vi "Get SMO RC Type.vi"(8 "error in (no error)":errorcluster, 11 "Inst.MagnetoInstrument in":refnum<class "Inst.Magneto.lvclass">) -> (0 "error out":errorcluster, 2 "Configuration.SMO.RC Type":T1=enum."STM", 3 "Inst.MagnetoInstrument out":refnum<class "Inst.Magneto.lvclass">)   [LabVIEW 2019, in "Inst.Magneto.lvclass"]
uses:
  Inst.Magneto.lvclass
  <userlib>/Levylab/Instrument Framework/SMOs/RemoteControl/Typedefs/RC Com Type--enum.ctl
  <userlib>/Levylab/Instrument Framework/Instrument Types/VSource/Instrument.VSource.lvclass
  <userlib>/Levylab/Instrument Framework/SMOs/RemoteControl/RemoteControl.lvclass
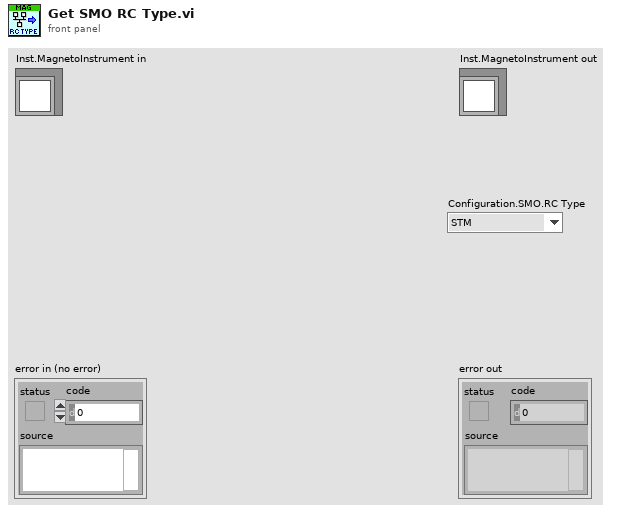
[diagram p1: front panel]
types:
  T1 = typedef "RemoteControl.lvclass/RC Com Type--enum.ctl" = enum16{"RC", "STM", "ZMQ"}
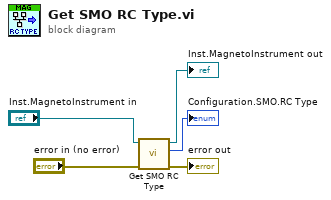
[diagram p0: block diagram]
diagram:
  n1 = call-parent "Get SMO RC Type.vi"("error in (no error)"="error in (no error)", "Instrument in"="Inst.MagnetoInstrument in") -> ("error out"=→"error out":errorcluster, "RC Type"=→"Configuration.SMO.RC Type":T1, "Instrument out"=→"Inst.MagnetoInstrument out":refnum<class "Inst.Magneto.lvclass">)  [unwired: 7 in]
